vi "Get and Set Test.vi"() -> ()   [LabVIEW 2017]
uses:
  String Subset.vi
  Parsing/Parse Full Path or Item Name.vi
  Offset/Find Item Locations by Path.vi
  JSONtext.lvlib
panel:
  out "Array 2":string[](array[string])
  out "Passed":bool[](array[boolean])
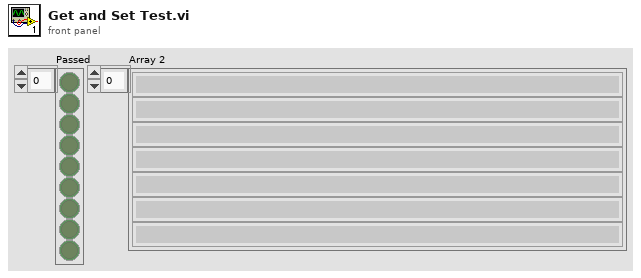
[diagram p1: front panel]
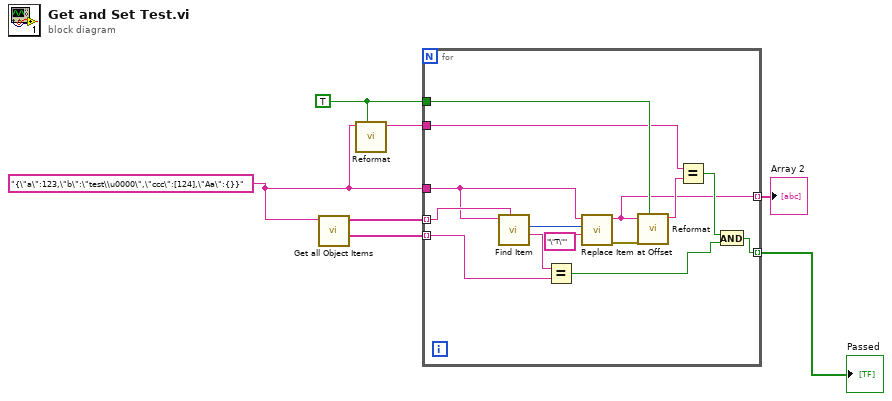
[diagram p0: block diagram]
diagram:
  w3 = TRUE ("Alphabetical Sort Objects")
  w4 = "{\"a\":123,\"b\":\"test\\u0000\",\"ccc\":[124],\"Aa\":{}}"
  n1 = call "Get all Object Items.vi"("JSON"=w4) -> ("<JSON>"=w7:string[], "Names"=w6:string[])  [unwired: 7 in, 2 out]
  n2 = call "Reformat.vi"("Alphabetical Sort Objects"=w3, "Input String"=w4) -> ("<JSON>First JSON Value"=w2:string)  [unwired: 6 in, 3 out]
  n3 = for {
    tunnel: w4 -> [w9]
    tunnel: w7 -> [w20] mode=indexing
    tunnel: w6 -> [w21] mode=indexing
    tunnel: [w12] -> w5 mode=indexing
    tunnel: w3 -> [w17]
    tunnel: w2 -> [w15]
    tunnel: [w11] -> w1 mode=indexing
    n4 = call "Find Item.vi"("$Path or Item Name"=w21, "JSON"=w9) -> ("<JSON>Item"=w19:string, "Item offset"=w8:i32)  [unwired: 6 in, 2 out]
    n5 = Equal?(x=w19, y=w20) -> (x = y?=w14:bool)
    n6 = call "Replace Item at Offset.vi"("<JSON>New Item"="\"T\"" ("JSON to Insert"), "Offset of Item to Replace"=w8, "<JSON> in"=w9) -> ("error out"=w18:errorcluster, "<JSON>"=w11:string)  [unwired: 7 in]
    n7 = call "Reformat.vi"("Alphabetical Sort Objects"=w17, "error in (no error)"=w18, "Input String"=w11) -> ("<JSON>First JSON Value"=w16:string)  [unwired: 5 in, 3 out]
    n8 = Equal?(x=w15, y=w16) -> (x = y?=w13:bool)
    n9 = And(x=w13, y=w14) -> (x .and. y?=w12:bool)
  }
  "Passed" <- w5
  "Array 2" <- w1
